vi "PH_Sound.PC Timing 3.vi"(0 "i ref in":refnum<vi>, 5 "error IO":errorcluster) -> (14 "i ref out":refnum<vi>, 19 "error out":errorcluster)   [LabVIEW 2014, in "PH_Sound.lvlib"]
doc: "This is a certain proc case."
uses:
  PH_Sound.lvlib
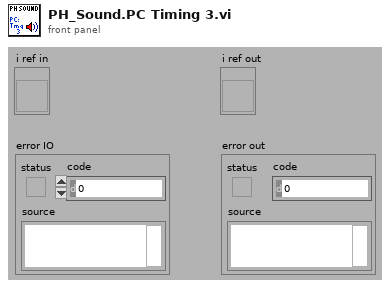
[diagram p1: front panel]
types:
  T1 = typedef "PH_Sound.lvlib/PH_Sound.i attribute.ctl" = cluster{"GUI Refs":cluster{"Exit":refnum<vi>, "Laserfreigabe":refnum<vi>, "PreAmp-Freigabe":refnum<vi>, "Countdown Running":refnum<vi>, "Emergency Off":refnum<vi>, "Device Error":refnum<vi>}, "Testalarm on":bool, "State":cluster{"Laser Class 4":bool, "PreAmp Running":bool, "Countdown Running":bool, "Emergency Off":bool}, "Starting Time":timestamp}
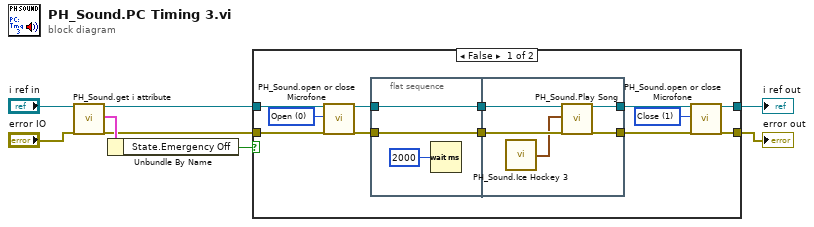
[diagram p0: block diagram]
diagram:
  n1 = call "PH_Sound.get i attribute.vi"("i ref in"="i ref in", "error in (no error)"="error IO") -> ("i ref out"=w2:refnum<vi>, "i attribute"=w3:T1, "error out"=w1:errorcluster)  [unwired: 15 in]
  n2 = Unbundle By Name(w3) -> ("State.Emergency Off"=w6:bool)
  n3 = case shown="False" w6 {
    tunnel: [w16 w30] -> w8
    tunnel: [w17 w29] -> w7
    tunnel: w1 -> [w19 w29]
    tunnel: w2 -> [w20 w30]
    frame False {
      w15 = u16 1 items=["Open", "Close"] ("Action")
      w18 = u16 0 items=["Open", "Close"] ("Action")
      n4 = call "PH_Sound.open or close Microfone.vi"("i ref in"=w20, "Action"=w18, "error in (no error)"=w19) -> ("i ref out"=w11:refnum<vi>, "error out"=w12:errorcluster)  [unwired: 15 in]
      n5 = flat-sequence {
        tunnel: w11 -> [w22]
        tunnel: w12 -> [w23]
        tunnel: [w23] -> w10
        tunnel: [w22] -> w9
        tunnel: [w28] -> w14
        tunnel: [w27] -> w13
        tunnel: w10 -> [w26]
        tunnel: w9 -> [w25]
        frame #0 {
          n6 = Wait (ms)(milliseconds to wait=u32 2000) -> ()  [unwired: 1 out]
        }
        frame #1 {
          n7 = call "PH_Sound.Ice Hockey 3.vi"() -> ("Ice Hockey 3"=w24:cluster{"Tone":dbl, "Beats":i32}[])  [unwired: 1 in]
          n8 = call "PH_Sound.Play Song.vi"("i ref in"=w25, "Song"=w24, "error in (no error)"=w26) -> ("i ref out"=w27:refnum<vi>, "error out"=w28:errorcluster)  [unwired: 15 in]
        }
      }
      n9 = call "PH_Sound.open or close Microfone.vi"("i ref in"=w13, "Action"=w15, "error in (no error)"=w14) -> ("i ref out"=w16:refnum<vi>, "error out"=w17:errorcluster)  [unwired: 15 in]
    }
    frame True {
    }
  }
  "i ref out" <- w8
  "error out" <- w7
